vi "Example_HVI_DIO.vi"() -> ()   [LabVIEW 2013]
uses:
  Instance           6 23Saved   Example_HVI_DIO .vi
panel:
  out "VI Path":string
  in  "Var11:":i32=6
  in  "Var10:":i32=47
  out "Var4=>":i32
  out "Var3=>":i32
  in  "Finish Program":bool
  out "Var=>\nHVIrunning":i32
  in  "Number variable\nHVI runinng":i32
  out "Port A Value (Hex)":i64 format="%08x"
  out "Bus In 0 value":i64
  out "cycle Count":i32
  out "Get HVI-Module Status":errorcluster
  out "HVI open Status":errorcluster
  in  "Module name in HVI":string="DIO"
  out "Close HVI Status":errorcluster
  in  "HVI file":string="Example_HVI_DIO.HVI"
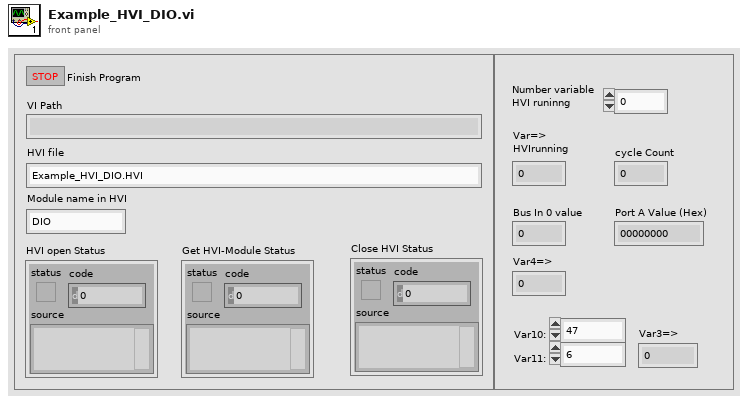
[diagram p1: front panel]
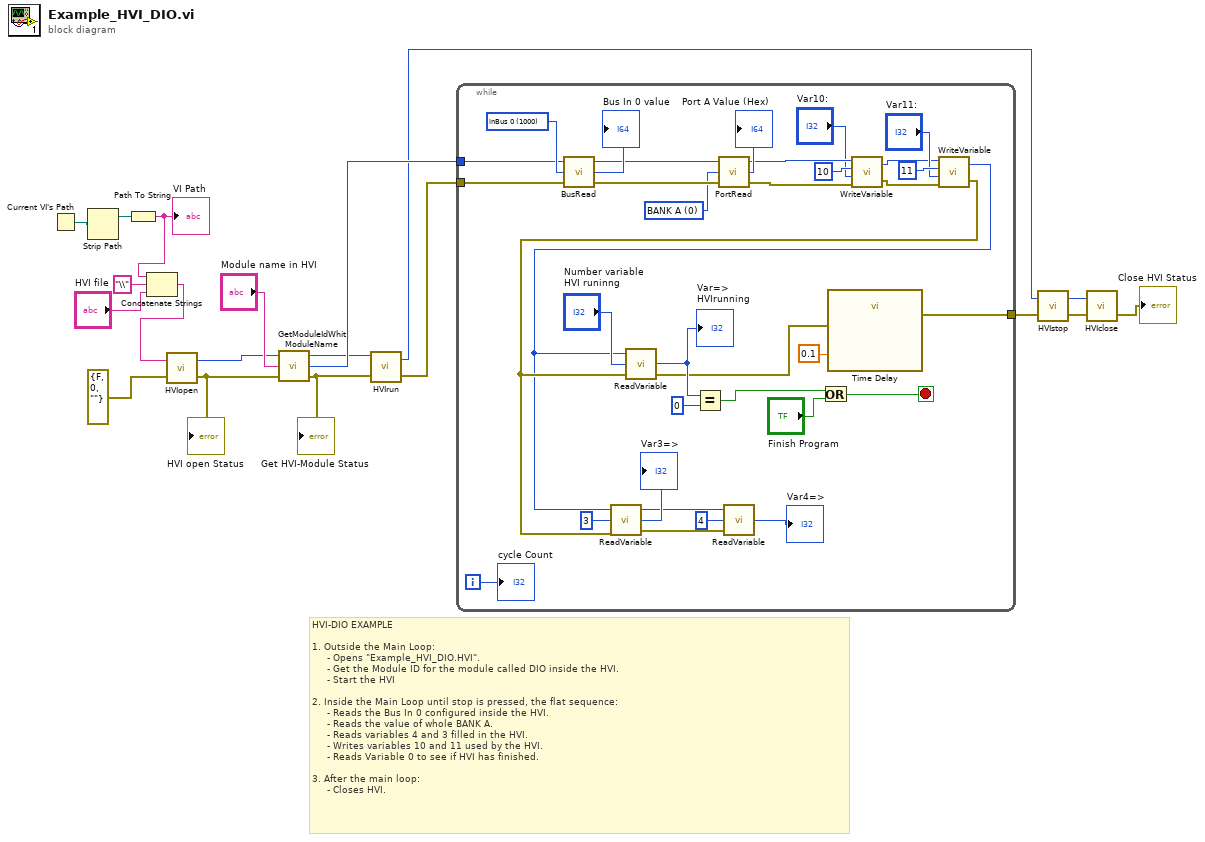
[diagram p0: block diagram]
diagram:
  # "HVI-DIO EXAMPLE\n\n1. Outside the Main Loop:\n     - Opens \"Example_HVI_DIO.HVI\".\n     - Get the Module ID for the module called DIO inside the HVI.\n     - Start the HVI\n\n2. Inside the Main Loop until stop is pressed, the flat sequence:\n     - Reads the Bus In 0 configured inside the HVI.\n     - Reads the value of whole BANK A.\n     - Reads variables 4 and 3 filled in the HVI.\n     - Writes variables 10 and 11 used by the HVI.\n     - Reads Variable 0 to see if HVI has finished.\n\n3. After the main loop:\n     - Closes HVI."
  n1 = Current VI's Path() -> (path=w11:path)
  n2 = Strip Path(path=w11) -> (stripped path=w10:path)  [unwired: 1 out]
  n3 = Path To String(path=w10) -> (string=w9:string)
  "VI Path" <- w9
  n4 = Concatenate Strings(w9, "\\" ("string"), "HVI file") -> (w7:string)
  n5 = call <vilib>:"HVIopen.vi"("errorIn"=errorcluster {"status"=FALSE, "code"=0, "source"=""}, "HVIfile"=w7) -> ("errorOut"=w5:errorcluster, "HVIID"=w4:i32)
  "HVI open Status" <- w5
  n6 = call <vilib>:"GetModuleIdWhitModuleName.vi"("errorIn"=w5, "ModuleName"="Module name in HVI", "HVIID"=w4) -> ("errorOut"=w16:errorcluster, "ModuleID"=w18:u32, "HVIIDOut"=w17:i32)
  "Get HVI-Module Status" <- w16
  n7 = call <vilib>:"HVIrun.vi"("errorIn"=w16, "HVIID"=w17) -> ("errorOut"=w15:errorcluster, "HVIIDOut"=w13:i32)
  n8 = while {
    tunnel: w18 -> [w46]
    tunnel: w15 -> [w45]
    tunnel: [w36] -> w14
    i -> [w47]
    stop <- w39 stop-if-true
    w48 = 0 items=["BANK A"=0, "BANK B"=1, "BANK B:A"=3000] ("nPort")
    w52 = 1000 items=["inBus 0"=1000] ("nInBus")
    n9 = call <vilib>:"BusRead.vi"("errorIn"=w45, "inBus"=w52, "moduleID"=w46) -> ("errorOut"=w49:errorcluster, "portValue"=→"Bus In 0 value":i64, "moduleIDOut"=w50:i32)
    n10 = call <vilib>:"PortRead.vi"("errorIn"=w49, "nPort"=w48, "moduleID"=w50) -> ("errorOut"=w26:errorcluster, "portValue"=→"Port A Value (Hex)":i64, "moduleIDOut"=w29:i32)
    n11 = call <vilib>:"WriteVariable.vi"("errorIn"=w26, "Value"="Var10:", "Number"=10 ("Number variable\nHVI runinng 3"), "ModuleID"=w29) -> ("errorOut"=w23:errorcluster, "ModuleIDOut"=w22:i32)
    n12 = call <vilib>:"WriteVariable.vi"("errorIn"=w23, "Value"="Var11:", "Number"=11 ("Number variable\nHVI runinng 3"), "ModuleID"=w22) -> ("errorOut"=w21:errorcluster, "ModuleIDOut"=w20:i32)
    n13 = call <vilib>:"ReadVariable.vi"("errorIn"=w21, "Number"=3 ("Number variable\nHVI runinng 2"), "ModuleID"=w20) -> ("errorOut"=w30:errorcluster, "variableValue"=→"Var3=>":i32, "ModuleIDOut"=w31:i32)
    n14 = call <vilib>:"ReadVariable.vi"("errorIn"=w21, "Number"="Number variable\nHVI runinng", "ModuleID"=w20) -> ("errorOut"=w37:errorcluster, "variableValue"=w43:i32)  [unwired: 1 out]
    "Var=>\nHVIrunning" <- w43
    n15 = Equal?(x=w43, y=0) -> (x = y?=w41:bool)
    n16 = call <vilib>:"ReadVariable.vi"("errorIn"=w30, "Number"=4 ("Number variable\nHVI runinng 3"), "ModuleID"=w31) -> ("variableValue"=→"Var4=>":i32)  [unwired: 2 out]
    n17 = Or(x=w41, y="Finish Program") -> (x .or. y?=w39:bool)
    n18 = call "Time Delay"("error in (no error)"=w37, "Delay Time (s)"=0.1) -> ("error out"=w36:errorcluster)  [unwired: 9 in]
    "cycle Count" <- w47
  }
  n19 = call <vilib>:"HVIstop.vi"("errorIn"=w14, "HVIID"=w13) -> ("errorOut"=w2:errorcluster, "HVIIDOut"=w1:i32)
  n20 = call <vilib>:"HVIclose.vi"("errorIn"=w2, "HVIID"=w1) -> ("errorOut"=→"Close HVI Status":errorcluster)  [unwired: 1 in]
